vi "Yscalingtest.vi"(6 "current":dbl, 8 "Nano Z Read":dbl, 9 "Current Maxed?":bool, 10 "Y":dbl, 11 "Plane Height":dbl) -> (3 "y scaled":dbl, 4 "Testoutput":dbl)   [LabVIEW 2017]
uses:
  <userlib>/HapticSTM/Feedbackless - Testdata/Zthreshholdtesting 2017 version/Zthreshholdtesting Folder/HapticSTM.lvlib
panel:
  out "force":cluster{"current":dbl}(graph)
  out "current":cluster{"current":dbl}(graph)
  out "Zpos":T1(graph)
  out "appended array":dbl[](array[numeric])
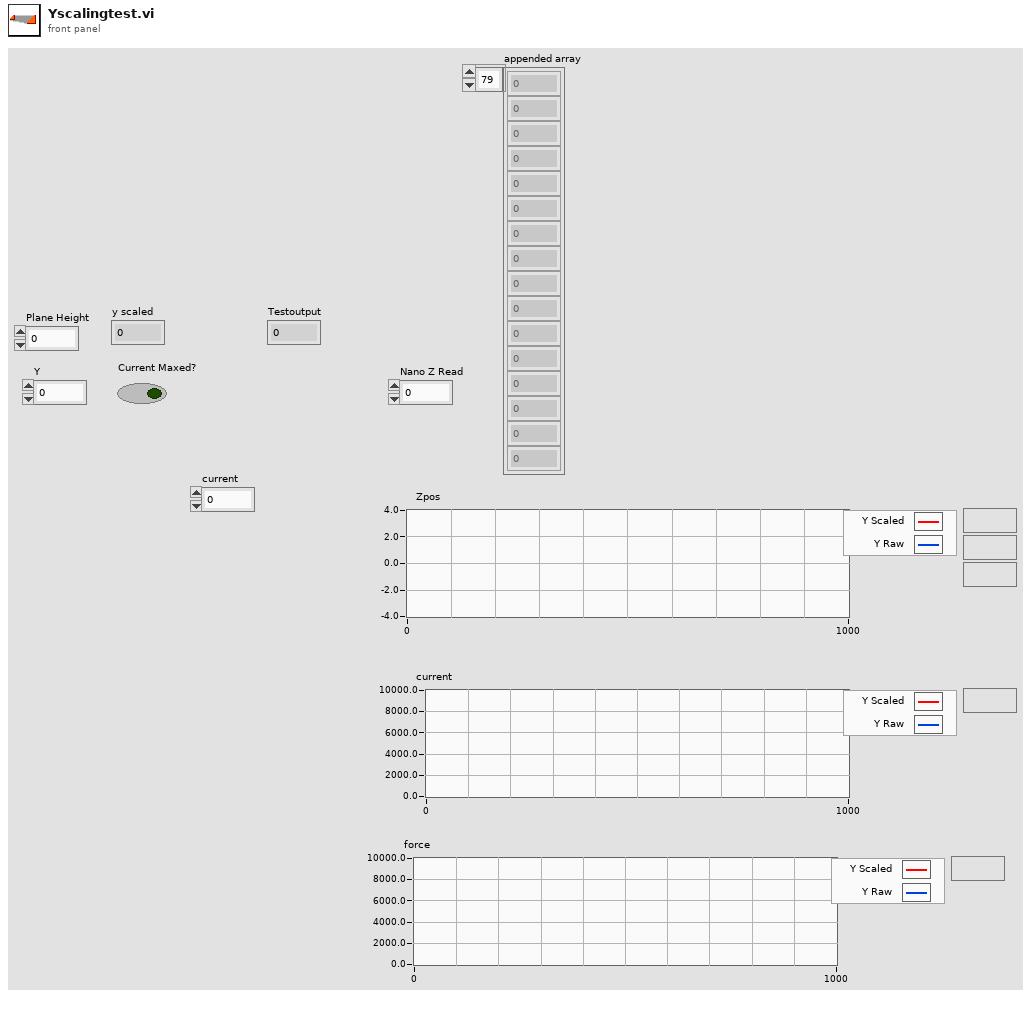
[diagram p1: front panel]
types:
  T1 = cluster{dbl, "function return":dbl, "function return":dbl}
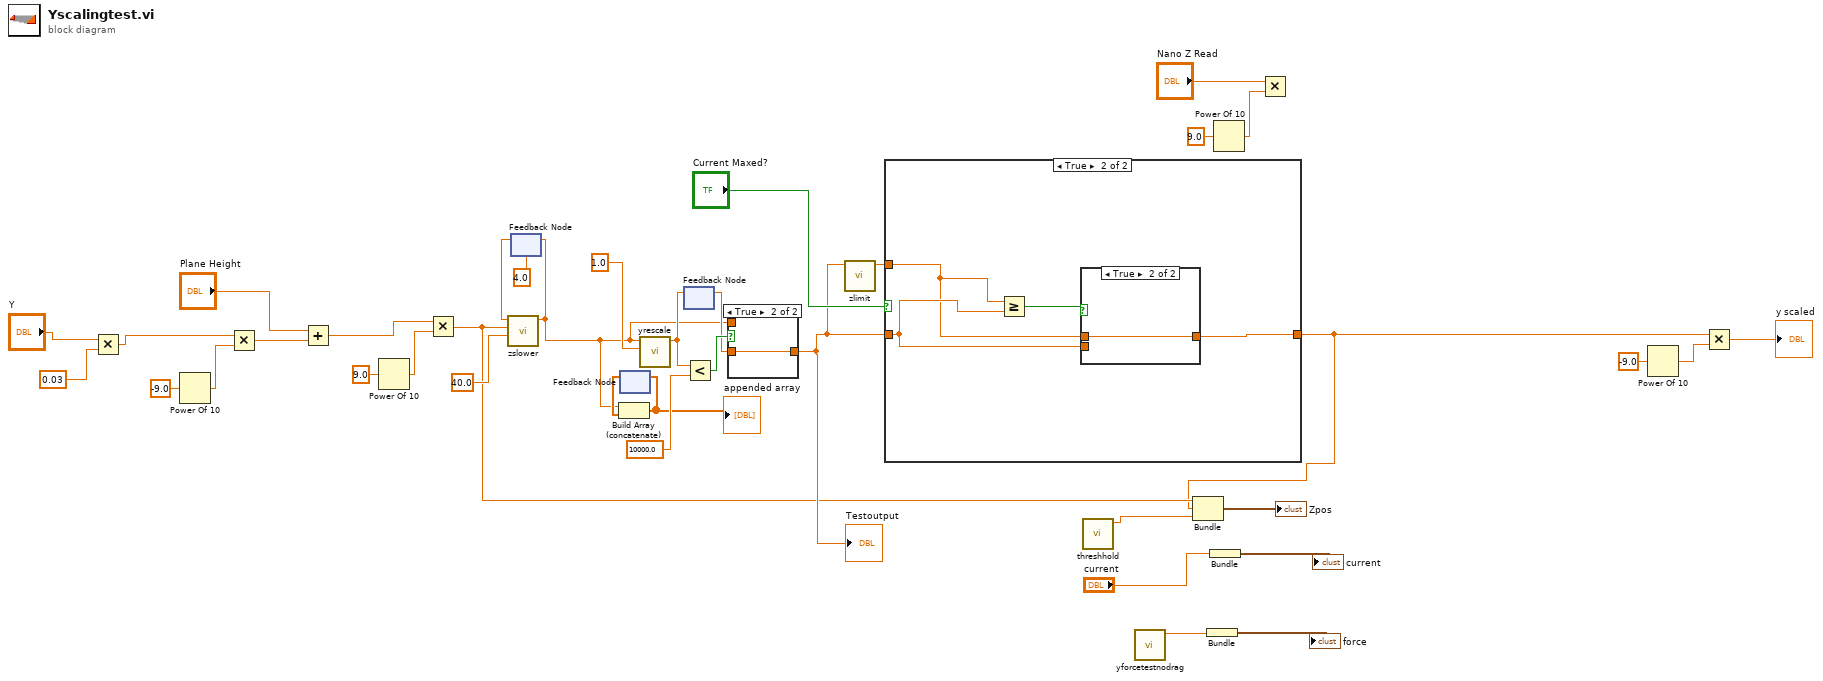
[diagram p0: block diagram]
diagram:
  n1 = Multiply(x="Y", y=0.03) -> (x*y=w34:dbl)
  n2 = Power Of 10(x=-9.0) -> (10^x=w33:dbl)
  n3 = Multiply(x=w34, y=w33) -> (x*y=w35:dbl)
  n4 = Add(x="Plane Height", y=w35) -> (x+y=w38:dbl)
  n5 = Power Of 10(x=9.0) -> (10^x=w37:dbl)
  n6 = Multiply(x=w38, y=w37) -> (x*y=w8:dbl)
  n7 = feedback #1(4.0 ("function return")) -> (w11:dbl)
  n8 = call <userlib>:"zslower.vi"("maxvel"=40.0, "labview_zpos_write"=w8, "nanonis_zpos_read"=w11) -> ("function return"=w10:dbl)  [unwired: 8 in]
  n9 = feedback-in #1(w10) -> ()
  n10 = feedback #2() -> (w13:dbl[])  [unwired: 1 in]
  n11 = Build Array (concatenate)(w10, w13) -> (w14:dbl[])
  "appended array" <- w14
  n12 = feedback-in #2(w14) -> ()
  n13 = call <userlib>:"yrescale.vi"("scalingfactor"=1.0, "ylabview"=w10) -> ("function return"=w19:dbl)  [unwired: 9 in]
  n14 = feedback-in #3(w19) -> ()
  n15 = feedback #3() -> (w18:dbl)  [unwired: 1 in]
  n16 = Less?(x=w19, y=10000.0) -> (x < y?=w20:bool)
  n17 = case shown="True" w20 {
    tunnel: [w39 w40] -> w22
    tunnel: w18 -> [_ w40]
    tunnel: w10 -> [w39 _]
    frame False {
    }
    frame True {
    }
  }
  "Testoutput" <- w22
  n18 = call <userlib>:"zlimit.vi"("yscaledinput"=w22) -> ("function return"=w23:dbl)  [unwired: 10 in]
  n19 = case shown="True" "Current Maxed?" {
    tunnel: [w41 w45] -> w7
    tunnel: w22 -> [w41 w43]
    tunnel: w23 -> [_ w42]
    frame False {
    }
    frame True {
      n20 = Greater Or Equal?(x=w42, y=w43) -> (x >= y?=w44:bool)
      n21 = case shown="True" w44 {
        tunnel: w42 -> [_ w47]
        tunnel: [w46 w47] -> w45
        tunnel: w43 -> [w46 _]
        frame False {
        }
        frame True {
        }
      }
    }
  }
  n22 = call <userlib>:"threshhold.vi"() -> ("function return"=w5:dbl)  [unwired: 11 in]
  n23 = call <userlib>:"yforcetestnodrag.vi"() -> ("function return"=w1:dbl)  [unwired: 11 in]
  n24 = Bundle(w8, "function return"=w7, "function return"=w5) -> (→"Zpos":T1)  [unwired: 1 in]
  n25 = Bundle("function return"=w1) -> (→"force":cluster{"function return":dbl})  [unwired: 1 in]
  n26 = Bundle("current"="current") -> (→"current":cluster{"current":dbl})  [unwired: 1 in]
  n27 = Power Of 10(x=9.0) -> (10^x=w17:dbl)
  n28 = Multiply(x="Nano Z Read", y=w17) -> ()  [unwired: 1 out]
  n29 = Power Of 10(x=-9.0) -> (10^x=w26:dbl)
  n30 = Multiply(x=w7, y=w26) -> (x*y=→"y scaled":dbl)
